vi "TrigClassworkMarcoGonzalez.vi"() -> ()   [LabVIEW 2012]
doc: "This VI will utilize a case structure with enums and rings to allow the user to find the sine, cosine, or tangent side of an angle."
panel:
  out "?":dbl
  in  "?":bool
  out "?":string
  in  "Trig Function":u16(ring) items=["Tangent", "Cosine", "Sine"]
  in  "Angle (Degrees)":dbl
  # "Marco Gonzalez\n02/06/2017\nEA3"
  # "="
  # "of"
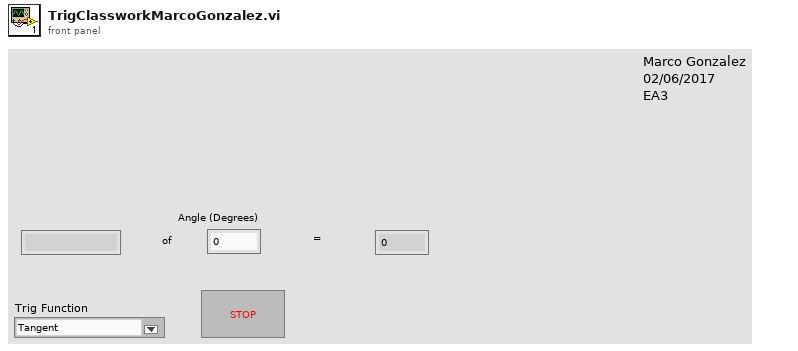
[diagram p1: front panel]
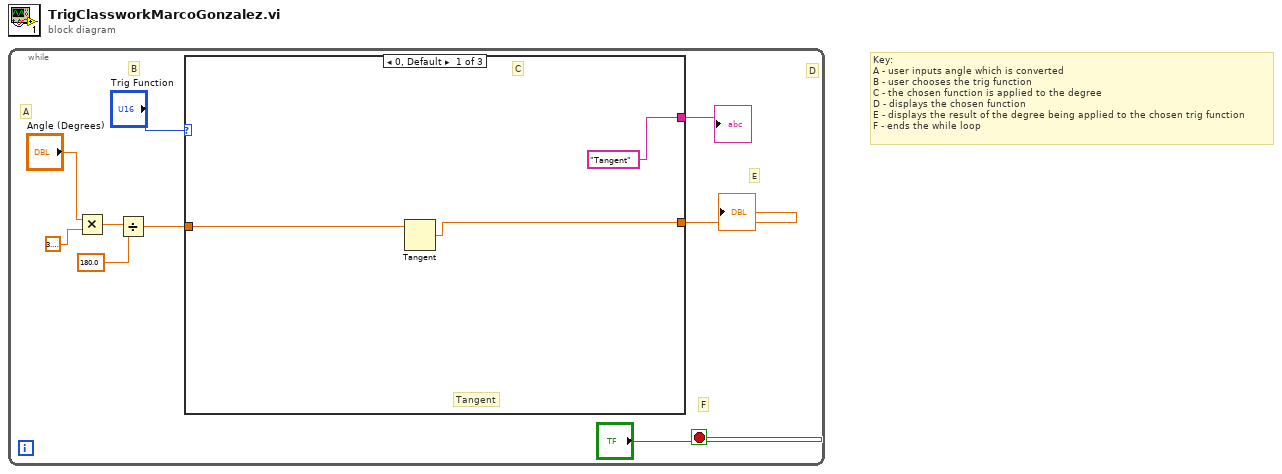
[diagram p0: block diagram]
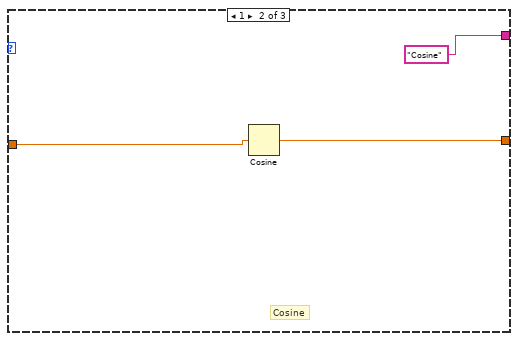
[diagram p2: hidden frame]
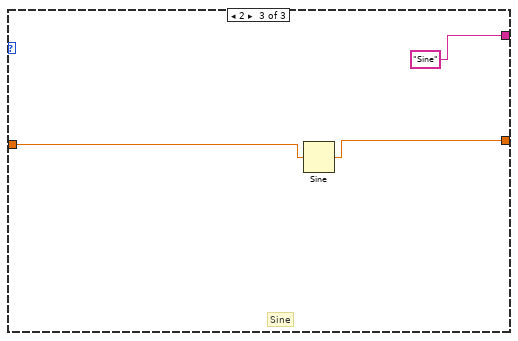
[diagram p3: hidden frame]
diagram:
  # "Key: \nA - user inputs angle which is converted\nB - user chooses the trig function\nC - the chosen function is applied to the degree\nD - displays the chosen function\nE - displays the result of the degree being applied to the chosen trig function\nF - ends the while loop"
  n1 = while {
    stop <- "?" stop-if-true
    # "F"
    # "E"
    # "D"
    # "B"
    # "A"
    n2 = Multiply(x="Angle (Degrees)", y=3.141592653589793) -> (x*y=w4:dbl)
    n3 = Divide(x=w4, y=180.0) -> (x/y=w2:dbl)
    n4 = case shown="0, Default" "Trig Function" {
      tunnel: ["Tangent" "Cosine" "Sine"] -> w8
      tunnel: w2 -> [w11 w14 w17]
      tunnel: [w10 w13 w16] -> w1
      frame 0, Default {
        # "C"
        # "Tangent"
        n5 = Tangent(1:w11) -> (0:w10:dbl)
      }
      frame 1 {
        # "Cosine"
        n6 = Cosine(x=w14) -> (cos(x)=w13:dbl)
      }
      frame 2 {
        # "Sine"
        n7 = Sine(x=w17) -> (sin(x)=w16:dbl)
      }
    }
    "?" <- w8
    "?" <- w1
  }
